vi "Arbitrary Feed Forward Generator.vi"(10 "Feed Forward Constants":cluster{"kA":dbl, "kS":dbl, "kG":dbl, "kV":dbl}={"kA"=0.0, "kS"=0.0, "kG"=-1.13, "kV"=0.0}, 11 "Setpoint":dbl) -> (3 "Arbitrary Feedforward":dbl)   [LabVIEW 2023]
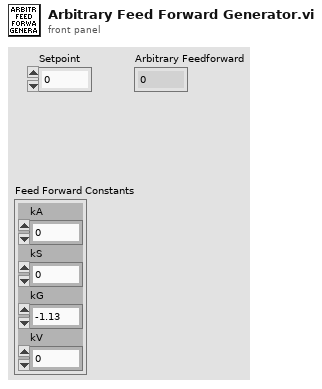
[diagram p1: front panel]
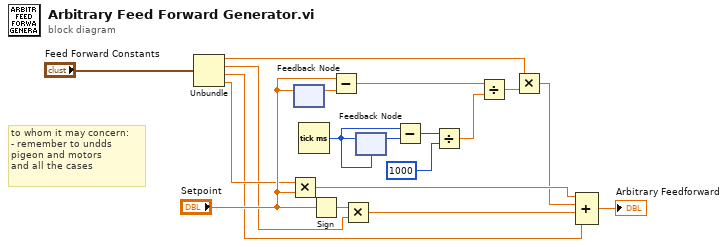
[diagram p0: block diagram]
diagram:
  # "to whom it may concern:\n- remember to undds\npigeon and motors\nand all the cases"
  n1 = Unbundle("Feed Forward Constants") -> ("kA"=w14:dbl, "kS"=w15:dbl, "kG"=w16:dbl, "kV"=w17:dbl)
  n2 = Multiply(x=w17, y="Setpoint") -> (x*y=w19:dbl)
  n3 = feedback #1() -> (w4:dbl)  [unwired: 1 in]
  n4 = feedback-in #1("Setpoint") -> ()
  n5 = Tick Count (ms)() -> (millisecond timer value=w7:u32)
  n6 = Sign(1:"Setpoint") -> (0:w2:dbl)
  n7 = Subtract(x="Setpoint", y=w4) -> (x-y=w5:dbl)
  n8 = Multiply(x=w2, y=w15) -> (x*y=w3:dbl)
  n9 = feedback #2(w7) -> (w6:u32)
  n10 = feedback-in #2(w7) -> ()
  n11 = Subtract(x=w7, y=w6) -> (x-y=w8:u32)
  n12 = Divide(x=w8, y=u32 1000) -> (x/y=w10:dbl)
  n13 = Divide(x=w5, y=w10) -> (x/y=w11:dbl)
  n14 = Multiply(x=w14, y=w11) -> (x*y=w12:dbl)
  n15 = Compound Arithmetic op=ADD(w19, w12, w3, w16) -> (→"Arbitrary Feedforward":dbl)
